vi "BNC_Initializer.vi"(11 "BNC Control Queue in":refnum<queue>) -> ()   [LabVIEW 2013]
uses:
  Hardware/BNC(QuantumComposers)/BNC_States.ctl
  <instrlib>/BNC/Public/BNC_Configs.ctl
  ControlDef/InstrumentSpecificControls/UIC-AToF/InitializationParams_BNC565_2Ch_AToF.ctl
  Hardware/BNC(QuantumComposers)/Command/Set C-Input.ctl
  Hardware/BNC(QuantumComposers)/Command/Set C-Mode.ctl
  Hardware/BNC(QuantumComposers)/Command/Set C-Output.ctl
  Hardware/BNC(QuantumComposers)/Command/Set C-Enable.ctl
panel:
  in  "BNC_Config":T1={"System"={"Rep.Rate"=1000.0, "Sys Ext Mode"=enum."Triggered", "Mode"=enum."Single Shot"}, "Channels"=[]}
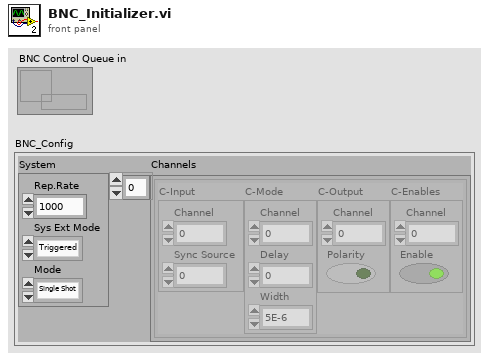
[diagram p1: front panel]
types:
  T1 = typedef "BNC_Configs.ctl" = cluster{"System":cluster{"Rep.Rate":dbl, "Sys Ext Mode":enum16{"Disabled", "Triggered", "Gated", "Triggered & Gated"}, "Mode":enum16{"Normal", "Single Shot", "Duty Cycle", "Burst"}}, "Channels":T2[]}
  T2 = typedef "InitializationParams_BNC565_2Ch_AToF.ctl" = cluster{"C-Input":T3, "C-Mode":T4, "C-Output":T5, "C-Enables":T6}
  T3 = typedef "Set C-Input.ctl" = cluster{"Channel":i32, "Sync Source":i32}
  T4 = typedef "Set C-Mode.ctl" = cluster{"Channel":i32, "Delay":dbl, "Width":dbl}
  T5 = typedef "Set C-Output.ctl" = cluster{"Channel":i32, "Polarity":bool}
  T6 = typedef "Set C-Enable.ctl" = cluster{"Channel":i32, "Enable":bool}
  T7 = typedef "BNC_States.ctl" = cluster{"State":enum16{"Initialize", "Set System", "Set C-Input", "Set C-Mode", "Set C-Output", "Set C-Enable", "Manl_Trig", "Run", "Stop", "Query C Number", "Close", "Quit"}, "Para.":variant}
  T8 = cluster{"Rep.Rate":dbl, "Sys Ext Mode":enum16{"Disabled", "Triggered", "Gated", "Triggered & Gated"}, "Mode":enum16{"Normal", "Single Shot", "Duty Cycle", "Burst"}}
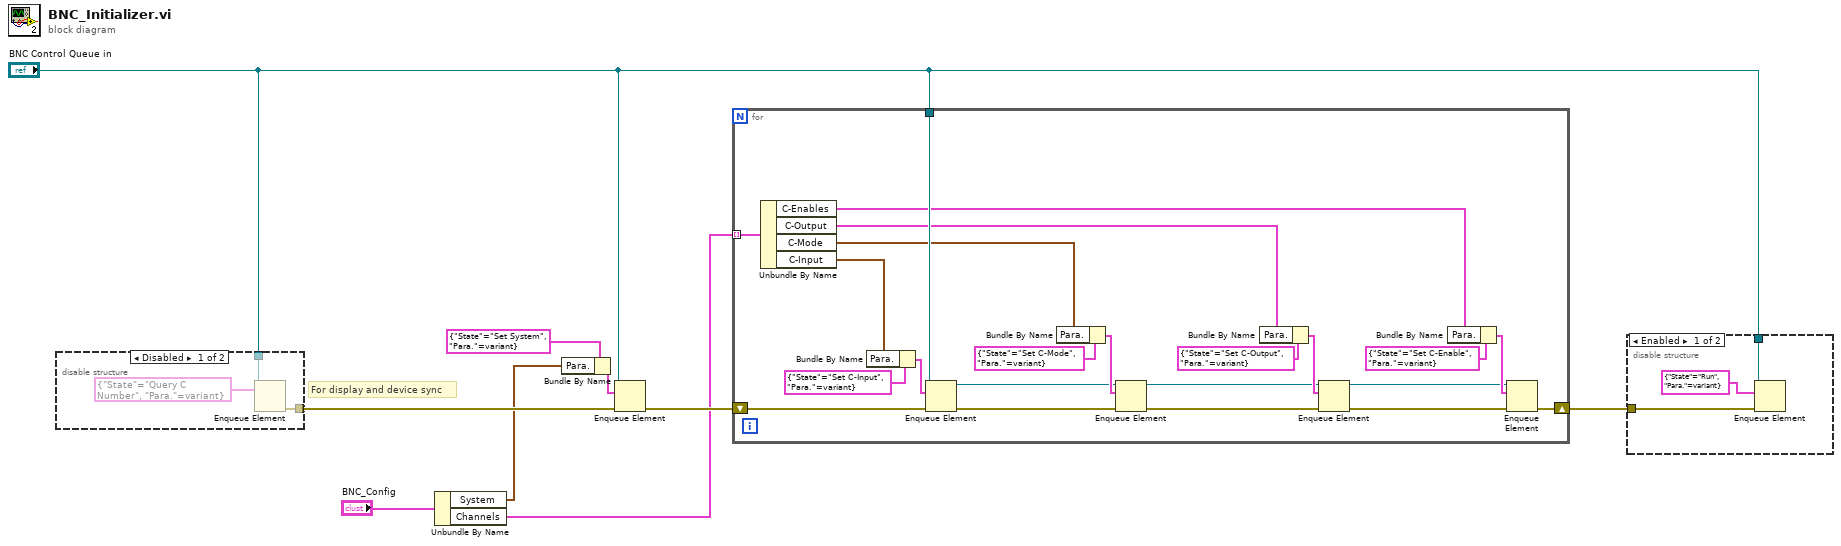
[diagram p0: block diagram]
diagram:
  # "For display and device sync"
  n1 = disable-structure shown="Disabled" {
    disable-tunnel: [w12 _] -> w6
    disable-tunnel: "BNC Control Queue in" -> [w10 _]
    frame Disabled {
      n2 = Enqueue Element(queue=w10, element=T7 {"State"=enum."Query C Number", "Para."=variant}) -> (error out=w12:errorcluster)  [unwired: 2 in, 2 out]
    }
    frame Enabled {
    }
  }
  n3 = Unbundle By Name("BNC_Config") -> ("System"=w1:T8, "Channels"=w3:T2[])
  n4 = Bundle By Name(cluster=T7 {"State"=enum."Set System", "Para."=variant} ("element"), "Para."=w1) -> (w8:T7)
  n5 = Enqueue Element(queue="BNC Control Queue in", element=w8, error in (no error)=w6) -> (error out=w9:errorcluster)  [unwired: 1 in, 2 out]
  n6 = for {
    tunnel: "BNC Control Queue in" -> [w31]
    tunnel: w3 -> [w30] mode=indexing
    shift-right: [w16] -> w5
    shift-left: w9 -> [w34]
    n7 = Unbundle By Name(w30) -> ("C-Enables"=w17:T6, "C-Output"=w18:T5, "C-Mode"=w19:T4, "C-Input"=w29:T3)
    n8 = Bundle By Name(cluster=T7 {"State"=enum."Set C-Input", "Para."=variant} ("element"), "Para."=w29) -> (w32:T7)
    n9 = Enqueue Element(queue=w31, element=w32, error in (no error)=w34) -> (queue out=w14:refnum<queue>, error out=w22:errorcluster)  [unwired: 1 in, 1 out]
    n10 = Bundle By Name(cluster=T7 {"State"=enum."Set C-Mode", "Para."=variant} ("element"), "Para."=w19) -> (w28:T7)
    n11 = Enqueue Element(queue=w14, element=w28, error in (no error)=w22) -> (queue out=w15:refnum<queue>, error out=w21:errorcluster)  [unwired: 1 in, 1 out]
    n12 = Bundle By Name(cluster=T7 {"State"=enum."Set C-Output", "Para."=variant} ("element"), "Para."=w18) -> (w25:T7)
    n13 = Enqueue Element(queue=w15, element=w25, error in (no error)=w21) -> (queue out=w13:refnum<queue>, error out=w20:errorcluster)  [unwired: 1 in, 1 out]
    n14 = Bundle By Name(cluster=T7 {"State"=enum."Set C-Enable", "Para."=variant} ("element"), "Para."=w17) -> (w24:T7)
    n15 = Enqueue Element(queue=w13, element=w24, error in (no error)=w20) -> (error out=w16:errorcluster)  [unwired: 1 in, 2 out]
  }
  n16 = disable-structure shown="Enabled" {
    disable-tunnel: w5 -> [w37 _]
    disable-tunnel: "BNC Control Queue in" -> [w36 _]
    frame Enabled {
      n17 = Enqueue Element(queue=w36, element=T7 {"State"=enum."Run", "Para."=variant}, error in (no error)=w37) -> ()  [unwired: 1 in, 3 out]
    }
    frame Disabled {
    }
  }
